vi "Send UI Reference.vi"(8 "error in (no error)":errorcluster, 9 "Name":string, 10 "VI Refnum":refnum<vi>, 11 "Chat Window UI Controller in":refnum<class "Chat Window UI Controller.lvclass">) -> (0 "error out":errorcluster, 3 "Chat Window UI Controller out":refnum<class "Chat Window UI Controller.lvclass">)   [LabVIEW 2015, in "Chat Window UI Controller.lvlib" / "Chat Window UI Controller.lvclass"]
uses:
  Chat Window UI Controller.lvclass
  <vilib>/ActorFramework/Actor/Actor.lvclass/Actor.ctl
  Chat Window UI Controller.lvclass/Chat Window UI Controller.ctl
  Chat Window UI Controller Messages/UI Panel Launched Msg/UI Panel Launched Msg.lvclass/UI Panel Launched Msg.ctl
  <vilib>/ActorFramework/Message Enqueuer/Message Enqueuer.lvclass/Message Enqueuer.ctl
  <vilib>/ActorFramework/Message Enqueuer/Enqueue.vi
  <vilib>/ActorFramework/Message Priority Queue/Priority Enqueue.vi
  Chat Window UI Controller Messages/UI Panel Launched Msg/UI Panel Launched Msg.lvclass
  <vilib>/ActorFramework/Actor/Actor.lvclass
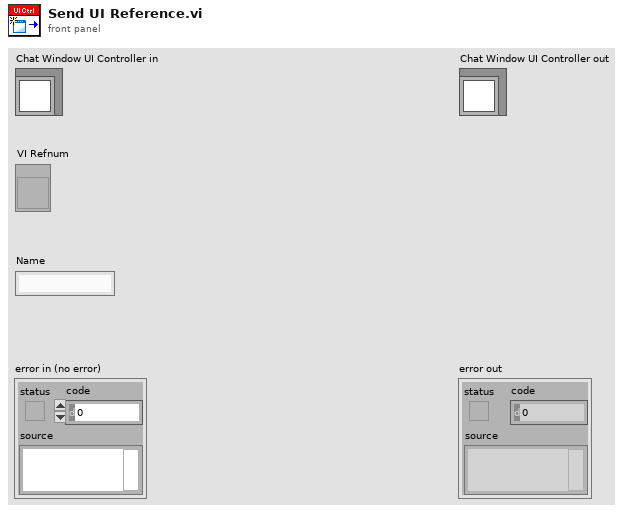
[diagram p1: front panel]
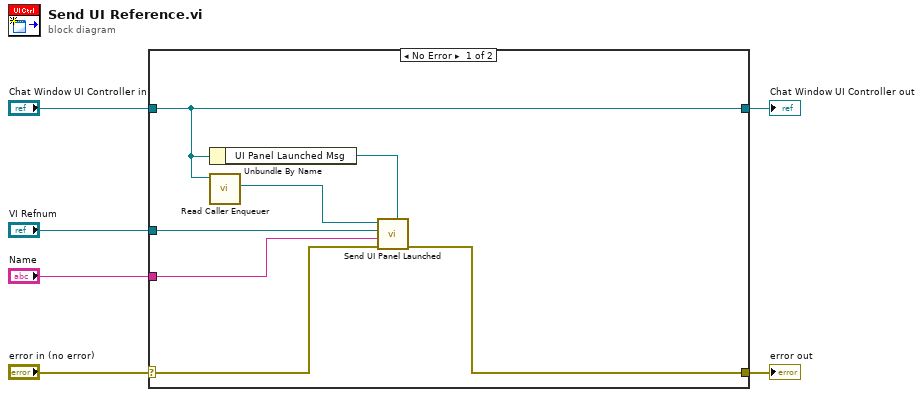
[diagram p0: block diagram]
diagram:
  n1 = case shown="No Error" "error in (no error)" {
    selector: "error in (no error)" -> [w8 w15]
    tunnel: [w7 w15] -> w5
    tunnel: [w12 w14] -> w3
    tunnel: "Chat Window UI Controller in" -> [w12 w14]
    tunnel: "VI Refnum" -> [w10 _]
    tunnel: "Name" -> [w9 _]
    frame No Error {
      n2 = Unbundle By Name(w12) -> ("UI Panel Launched Msg"=w13:refnum<class "UI Panel Launched Msg.lvclass">)
      n3 = call <vilib>:"Read Caller Enqueuer.vi"("Actor"=w12) -> ("Caller Enqueuer"=w11:refnum<class "Message Enqueuer.lvclass">)  [unwired: 10 in]
      n4 = call "Send UI Panel Launched.vi"("Message Type"=w13, "error in (no error)"=w8, "Name"=w9, "VI Refnum"=w10, "Message Enqueuer"=w11) -> ("error out"=w7:errorcluster)  [unwired: 5 in, 1 out]
    }
    frame Error {
    }
  }
  "error out" <- w5
  "Chat Window UI Controller out" <- w3
